vi "Set error.vi"(8 "error in (no error)":errorcluster, 11 "Control-Client in":refnum<class "Control-Client.lvclass">) -> (0 "error out":errorcluster, 3 "Control-Client out":refnum<class "Control-Client.lvclass">)   [LabVIEW 2015, in "Control-Client.lvclass"]
uses:
  Control-Client.lvclass
  GeneralFunctionality/GeneralFunctionality.lvclass/GeneralFunctionality.ctl
  GeneralFunctionality/GeneralFunctionality.lvclass
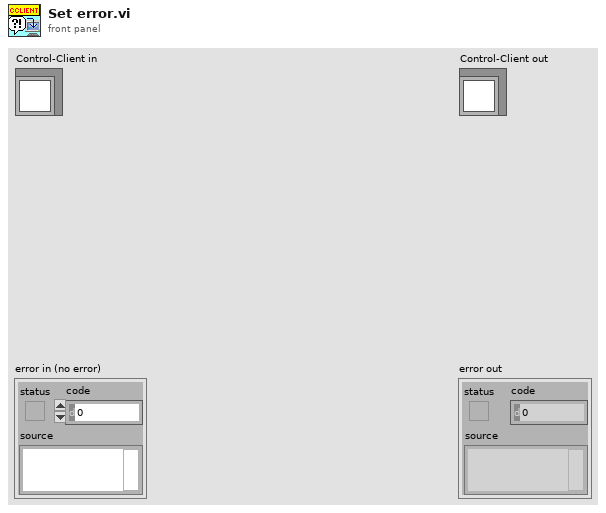
[diagram p1: front panel]
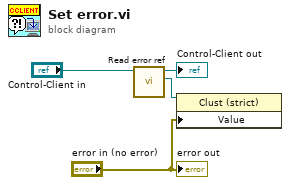
[diagram p0: block diagram]
diagram:
  n1 = call "Read error ref.vi"("GeneralFunctionality in"="Control-Client in") -> ("error"=w2:refnum<vi>, "GeneralFunctionality out"=→"Control-Client out":refnum<class "Control-Client.lvclass">)  [unwired: 8 in, 1 out]
  n2 = property class="Clust (strict)"(reference=w2, "Value"="error in (no error)") -> ()  [unwired: 1 in, 2 out]
  "error out" <- "error in (no error)"
